vi "Run System Exec Command.vi"() -> ()   [LabVIEW 2020]
panel:
  out "Array 2":string[](array[string])
  out "Numeric":i32
  out "Array":string[](array[string])
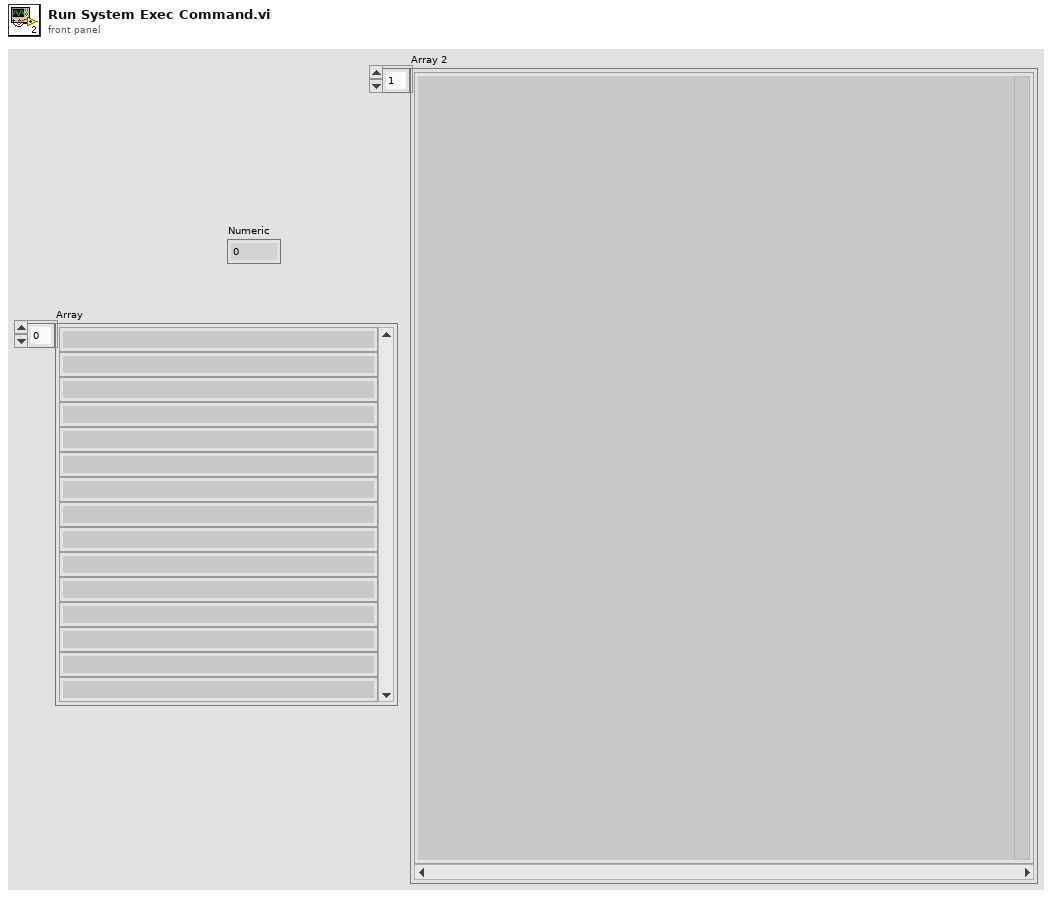
[diagram p1: front panel]
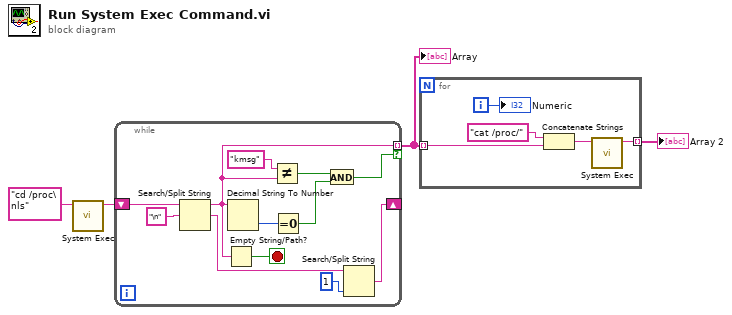
[diagram p0: block diagram]
diagram:
  n1 = call <vilib>:"System Exec.vi"("command line"="cd /proc\nls") -> ("standard output"=w3:string)  [unwired: 7 in, 3 out]
  n2 = while {
    tunnel: [w9] -> w2 mode=indexing if=w5
    shift-right: [w13] -> _
    shift-left: w3 -> [w15]
    stop <- w10 stop-if-true
    n3 = Search/Split String(string=w15, search string/char (-)="\n") -> (substring before match=w9:string, match + rest of string=w11:string)  [unwired: 1 in, 1 out]
    n4 = Empty String/Path?(string/path=w9) -> (empty?=w10:bool)
    n5 = Decimal String To Number(string=w9) -> (number=w12:i32)  [unwired: 2 in, 1 out]
    n6 = Not Equal?(x="kmsg" ("y"), y=w9) -> (x != y?=w6:bool)
    n7 = Equal To 0?(x=w12) -> (x = 0?=w7:bool)
    n8 = And(x=w6, y=w7) -> (x .and. y?=w5:bool)
    n9 = Search/Split String(string=w11, offset (0)=1) -> (match + rest of string=w13:string)  [unwired: 1 in, 2 out]
  }
  "Array" <- w2
  n10 = for {
    tunnel: w2 -> [w20] mode=indexing
    tunnel: [w18] -> w1 mode=indexing
    i -> [w17]
    n11 = Concatenate Strings("cat /proc/" ("string"), w20) -> (w19:string)
    n12 = call <vilib>:"System Exec.vi"("command line"=w19) -> ("standard output"=w18:string)  [unwired: 7 in, 3 out]
    "Numeric" <- w17
  }
  "Array 2" <- w1
